vi "Get Scalar Datatypes and Refs.vi"(8 "error in (no error)":errorcluster, 10 "Item GUID":string, 11 "Section Ref in":T5 format="%.0x") -> (0 "error out":errorcluster, 1 "Default Values":dbl[](array[numeric]), 2 "VS Ref":T5[](array[typedef]) format="%.0x", 3 "Section Ref out":T5 format="%.0x", 4 "Registers Ref":T1[](array[typedef]) {"Register"."Data Type" format="%.0x"})   [LabVIEW 2015, in "FPGA Addon System Explorer.lvlib"]
uses:
  FPGA Addon System Explorer.lvlib
  <vilib>/NI Veristand/Custom Device API/Custom Device Item Ref.ctl
  Shared/Compiled.RegisterSettings.ctl
  Shared/Scalar Type.ctl
  Shared/Register Information.ctl
  Shared/Data Type.ctl
  Shared/FG Action.ctl
  <vilib>/NI Veristand/Custom Device API/Get Item Property (String).vi
  <vilib>/NI Veristand/Custom Device API/NI VeriStand - Set Item Property.vi
  <vilib>/NI Veristand/Custom Device API/Set Item Property (Variant).vi
  <vilib>/NI Veristand/Custom Device API/Get Item Property (Variant).vi
  Shared/Constants.vi
  <vilib>/NI Veristand/Custom Device Tools/Custom Device Utility Library/NI VeriStand - Search for Item by GUID.vi
  <vilib>/NI VeriStand/Custom Device API/Custom Device API.lvlib
  <vilib>/NI VeriStand/Custom Device Tools/Custom Device Utility Library/Custom Device Utility Library.lvlib
  Shared/FPGA Addon Shared.lvlib
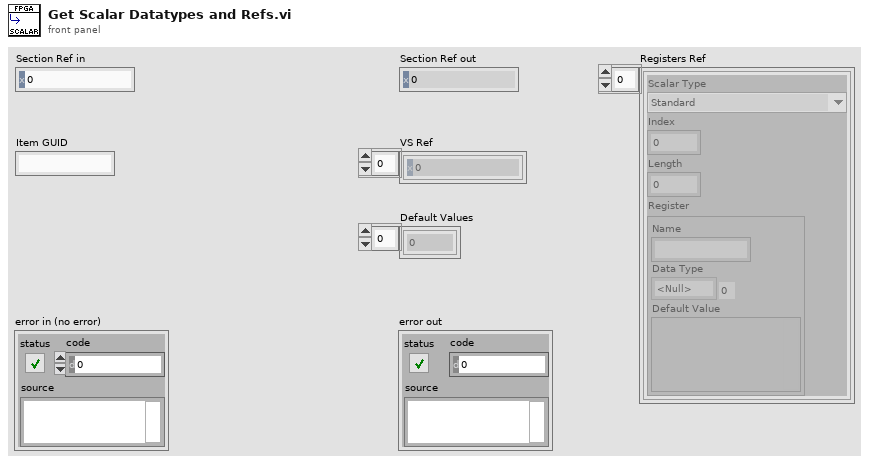
[diagram p1: front panel]
types:
  T1 = typedef "FPGA Addon Shared.lvlib/Compiled.RegisterSettings.ctl" = cluster{"Scalar Type":T2, "Index":i32, "Length":i32, "Register":T3}
  T2 = typedef "FPGA Addon Shared.lvlib/Scalar Type.ctl" = enum16{"Standard", "Bitpacked"}
  T3 = typedef "FPGA Addon Shared.lvlib/Register Information.ctl" = cluster{"Name":string, "Data Type":T4, "Default Value":variant}
  T4 = typedef "FPGA Addon Shared.lvlib/Data Type.ctl" = enum8{"<Null>", "I8", "I16", "I32", "I64", "U8", "U16", "U32", "U64", "SGL", "Boolean", "Analog PWM In Settings", "Analog PWM In", "Digital PWM In Settings", "Digital PWM In", "Digital PWM Out", "Sine Out", "FXP+/-24.5", "FXP+/-16.5", "FXP+/-32.8", "FXP+/-64.32", "FXP+/-16.7", "FXP+/-20.5", "FXP+/-27.5", "FXP+/-32.16", "Digital Static In", "Digital Static Out", "Digital Static In Settings", "Digital WSS Out"}
  T5 = typedef "Custom Device API.lvlib/Custom Device Item Ref.ctl" = u64
  T6 = typedef "FPGA Addon Shared.lvlib/FG Action.ctl" = enum8{"GET", "SET"}
  T7 = typedef "Custom Device API.lvlib/Custom Device Item Info.ctl" = cluster{"Name":string, "Is Channel":bool, "GUID":string, "Is Waveform":bool}
  T8 = typedef "Custom Device API.lvlib/Custom Device Channel.ctl" = cluster{"Type":T9, "Units":string, "Default Value":dbl, "Faultable":bool, "Scalable":bool}
  T9 = typedef "Custom Device API.lvlib/Custom Device Channel Type.ctl" = enum16{"Input", "Output"}
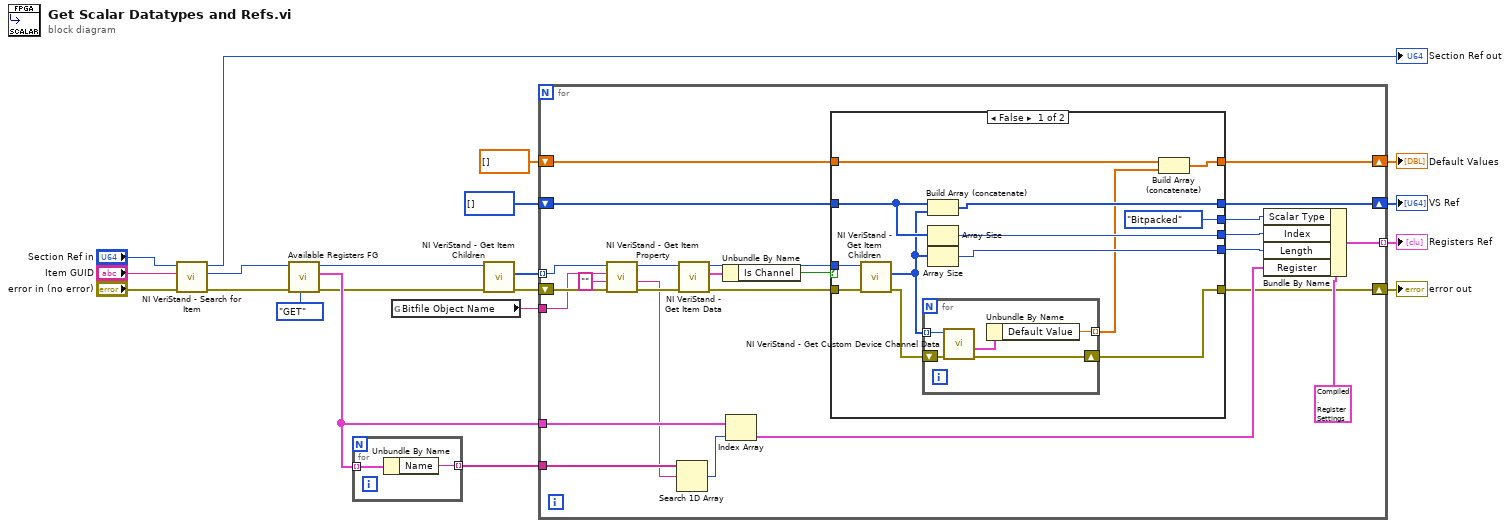
[diagram p0: block diagram]
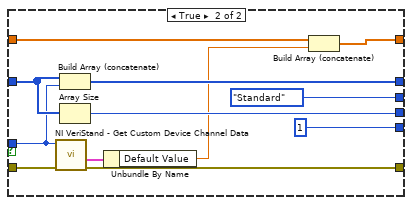
[diagram p2: hidden frame]
diagram:
  n1 = call-poly <vilib>:"NI VeriStand - Search for Item.vi"("error in"="error in (no error)", "Item GUID"="Item GUID", "Section Ref in"="Section Ref in") -> ("error out"=w19:errorcluster, "Item Ref"=w20:T5, "Section Ref out"=→"Section Ref out":T5)  [unwired: 5 in, 1 out]
  n2 = call "Available Registers FG.vi"("Action"=FG_Action."GET", "error in (no error)"=w19, "Item Ref"=w20) -> ("error out"=w16:errorcluster, "Available Registers"=w17:T3[], "Item Ref out"=w18:T5)  [unwired: 6 in]
  n3 = for {
    tunnel: w17 -> [w22] mode=indexing
    tunnel: [w21] -> w15 mode=indexing
    n4 = Unbundle By Name(w22) -> ("Name"=w21:string)
  }
  n5 = global read "Constants.vi" "Bitfile Object Name"() -> (w14:string)
  n6 = call <vilib>:"NI VeriStand - Get Item Children.vi"("error in (no error)"=w16, "Item Ref in"=w18) -> ("error out"=w12:errorcluster, "Child Refs"=w13:T5[])  [unwired: 6 in, 2 out]
  n7 = for {
    shift-right: [w25] -> w6
    shift-left: w12 -> [w47]
    tunnel: w13 -> [w46] mode=indexing
    tunnel: w14 -> [w45]
    tunnel: w15 -> [w43]
    tunnel: w17 -> [w41]
    shift-right: [w33] -> w4
    shift-left: T5[] [] -> [w34]
    tunnel: [w32] -> w5 mode=indexing
    shift-right: [w24] -> w1
    shift-left: dbl[] [] -> [w23]
    n8 = call-poly <vilib>:"NI VeriStand - Get Item Property.vi"("error in (no error)"=w47, "Default Value"="", "Property Name"=w45, "Item Ref in"=w46) -> ("error out"=w39:errorcluster, "Value"=w31:string, "Item Ref out"=w42:T5)  [unwired: 4 in, 1 out]
    n9 = Search 1D Array(1D array=w43, element=w31) -> (index of element=w40:i32)  [unwired: 1 in]
    n10 = call <vilib>:"NI VeriStand - Get Item Data.vi"("error in (no error)"=w39, "Item Ref in"=w42) -> ("error out"=w36:errorcluster, "Item Info"=w38:T7, "Item Ref out"=w37:T5)  [unwired: 6 in, 1 out]
    n11 = Unbundle By Name(w38) -> ("Is Channel"=w35:bool)
    n12 = Index Array(array=w41, index=w40) -> (element=w26:T3)
    n13 = case shown="False" w35 {
      tunnel: w37 -> [w59 w72]
      tunnel: w36 -> [w60 w71]
      tunnel: [w50 w70] -> w25
      tunnel: w34 -> [w57 w75]
      tunnel: [w58 w77] -> w33
      tunnel: [Scalar_Type."Bitpacked" ("Scalar Type") Scalar_Type."Standard" ("Scalar Type")] -> w30
      tunnel: [w56 w74] -> w29
      tunnel: [w55 1] -> w28
      tunnel: [w48 w67] -> w24
      tunnel: w23 -> [w52 w66]
      frame False {
        n14 = call <vilib>:"NI VeriStand - Get Item Children.vi"("error in (no error)"=w60, "Item Ref in"=w59) -> ("error out"=w51:errorcluster, "Child Refs"=w53:T5[])  [unwired: 6 in, 2 out]
        n15 = for {
          tunnel: w53 -> [w64] mode=indexing
          shift-right: [w62] -> w50
          shift-left: w51 -> [w63]
          tunnel: [w61] -> w49 mode=indexing
          n16 = call <vilib>:"NI VeriStand - Get Custom Device Channel Data.vi"("error in (no error)"=w63, "Channel Ref in"=w64) -> ("error out"=w62:errorcluster, "Channel"=w65:T8)  [unwired: 4 in, 4 out]
          n17 = Unbundle By Name(w65) -> ("Default Value"=w61:dbl)
        }
        n18 = Build Array (concatenate)(w57, w53) -> (w58:T5[])
        n19 = Array Size(array=w57) -> (size(s)=w56:i32)
        n20 = Array Size(array=w53) -> (size(s)=w55:i32)
        n21 = Build Array (concatenate)(w52, w49) -> (w48:dbl[])
      }
      frame True {
        n22 = call <vilib>:"NI VeriStand - Get Custom Device Channel Data.vi"("error in (no error)"=w71, "Channel Ref in"=w72) -> ("error out"=w70:errorcluster, "Channel"=w69:T8)  [unwired: 4 in, 4 out]
        n23 = Build Array (concatenate)(w75, w72) -> (w77:T5[])
        n24 = Array Size(array=w75) -> (size(s)=w74:i32)
        n25 = Unbundle By Name(w69) -> ("Default Value"=w68:dbl)
        n26 = Build Array (concatenate)(w66, w68) -> (w67:dbl[])
      }
    }
    n27 = Bundle By Name(cluster=T1 {"Scalar Type"=enum."Standard", "Index"=0, "Length"=0, "Register"={"Name"="", "Data Type"=enum."<Null>", "Default Value"=variant(dbl 0.0)}} ("Cluster"), "Scalar Type"=w30, "Index"=w29, "Length"=w28, "Register"=w26) -> (w32:T1)
  }
  "error out" <- w6
  "VS Ref" <- w4
  "Registers Ref" <- w5
  "Default Values" <- w1
